vi "全局 小时数据发送次数.vi"() -> ()   [LabVIEW 2016, in "数据传输系统.lvlib"]
panel:
  out "告警码":i32
  out "小时数据发送次数":i32
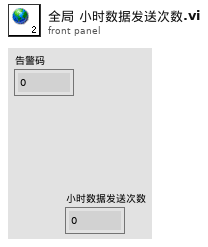
[diagram p1: front panel]
diagram:
